vi "getDescription.vi"(8 "error in (no error)":errorcluster, 11 "Vanilla in":refnum<class "Vanilla.lvclass">) -> (0 "error out":errorcluster, 2 "description":string, 3 "Vanilla out":refnum<class "Vanilla.lvclass">)   [LabVIEW 2017, in "Vanilla.lvclass"]
uses:
  Vanilla.lvclass
  CondimentDecorator/CondimentDecorator.lvclass
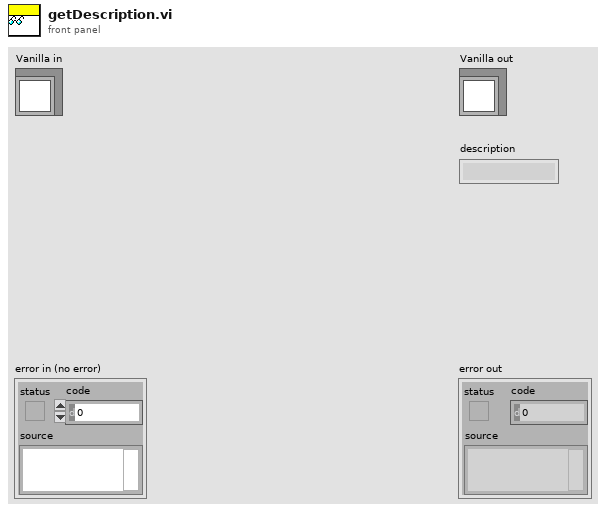
[diagram p1: front panel]
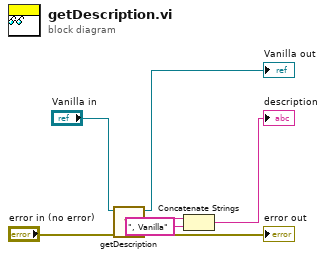
[diagram p0: block diagram]
diagram:
  n1 = call-parent "getDescription.vi"("error in (no error)"="error in (no error)", "CondimentDecorator in"="Vanilla in") -> ("error out"=→"error out":errorcluster, "description"=w6:string, "CondimentDecorator out"=→"Vanilla out":refnum<class "Vanilla.lvclass">)  [unwired: 7 in]
  n2 = Concatenate Strings(w6, ", Vanilla" ("string")) -> (→"description":string)
